vi "tcpMessageClient.vi"(11 "client configuration":T2={"client ID"="tcpClient", "remote host"="localhost", "local port"=50000, "remote port"=50001}) -> (0 "error out":errorcluster)   [LabVIEW 2014]
doc: "A couple tcpMessageServer and tcpMessageClient ensures communication between two instances. Each one can both transmit or receive CR/LF terminated message strings; however one of the member has to be a Server and the other a Client. Both sit and wait for the other party to connect.\n\nThe difference is: \n* the Server accpts connections on the specified port from any incoming host (the inputs \"remote host\" and \"remote port\" are ignored) \n* the Client must know to which host is directed\n\nCommunication with them, while running, is done via four named queues. One acts as a transmission buffer, another as a receive buffer; one is a single element queue, which cause the shutdown of the actor when a True is enqueued to it; the last one is a read only one-element queue which reports the actor status."
uses:
  typedefs/clientConfiguration.ctl
  typedefs/clientStatus.ctl
panel:
  out "status":T1
  out "received string":string
  out "string to send":string
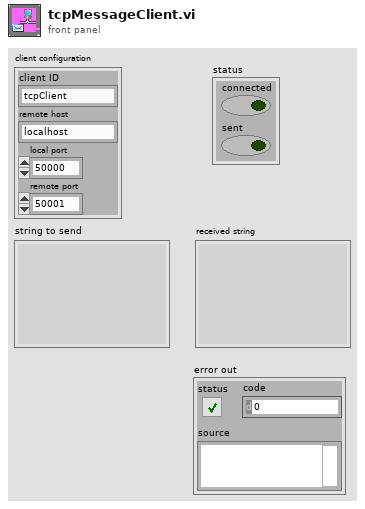
[diagram p1: front panel]
types:
  T1 = typedef "clientStatus.ctl" = cluster{"connected":bool, "sent":bool}
  T2 = typedef "clientConfiguration.ctl" = cluster{"client ID":string, "remote host":string, "local port":u16, "remote port":u16}
  T3 = cluster{"status":cluster{"queue":refnum<queue>, "error out":errorcluster}, "receive":cluster{"queue":refnum<queue>, "error out":errorcluster}, "transmit":cluster{"queue":refnum<queue>, "error out":errorcluster}, "shutdown":cluster{"queue":refnum<queue>, "error out":errorcluster}}
  T4 = cluster{"queue":refnum<queue>, "error out":errorcluster}
  T5 = enum16{"Standard", "Buffered", "CRLF", "Immediate"}
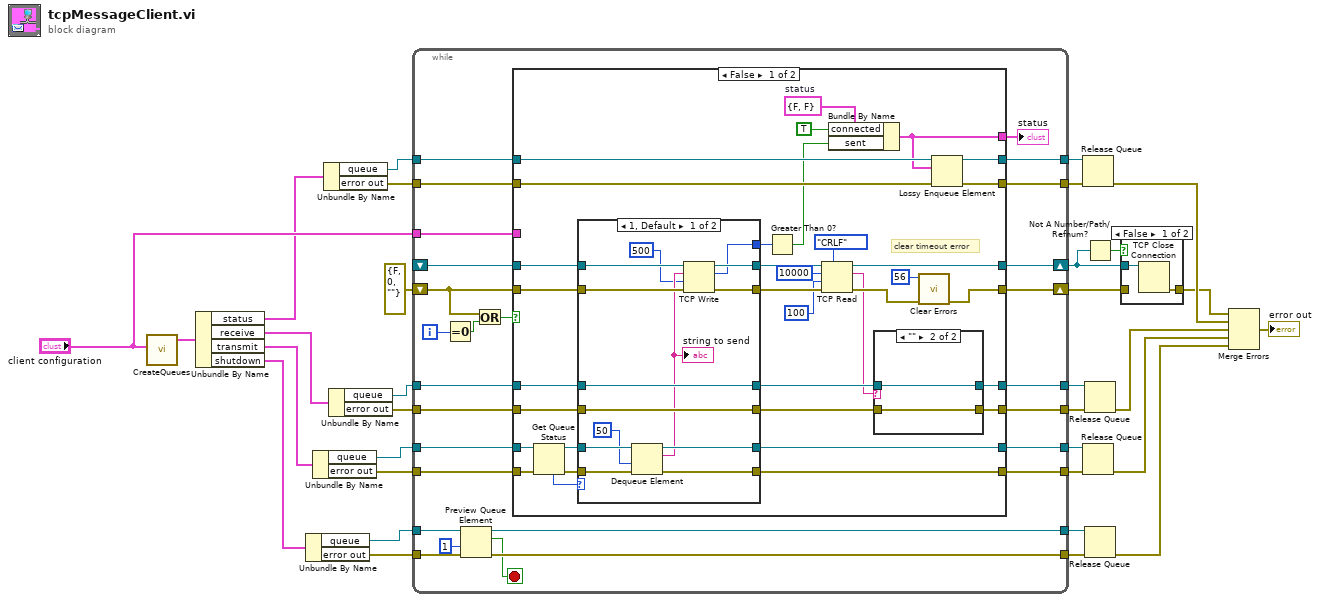
[diagram p0: block diagram]
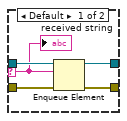
[diagram p3: hidden frame]
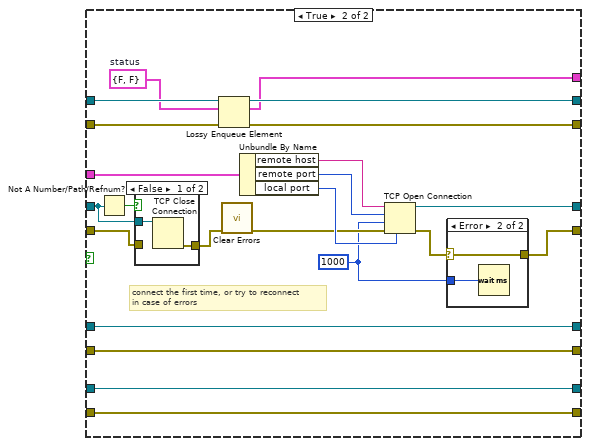
[diagram p5: hidden frame]
diagram:
  n1 = call "CreateQueues.vi"("client configuration"="client configuration") -> ("output cluster"=w5:T3)  [unwired: 10 in]
  n2 = Unbundle By Name(w5) -> ("status"=w8:T4, "receive"=w11:T4, "transmit"=w12:T4, "shutdown"=w17:T4)
  n3 = Unbundle By Name(w17) -> ("queue"=w16:refnum<queue>, "error out"=w15:errorcluster)
  n4 = Unbundle By Name(w12) -> ("queue"=w13:refnum<queue>, "error out"=w14:errorcluster)
  n5 = Unbundle By Name(w8) -> ("queue"=w7:refnum<queue>, "error out"=w6:errorcluster)
  n6 = Unbundle By Name(w11) -> ("queue"=w10:refnum<queue>, "error out"=w9:errorcluster)
  n7 = while {
    shift-right: [w57] -> w2
    shift-left: errorcluster {"status"=FALSE, "code"=0, "source"=""} ("error out") -> [w56]
    shift-right: [w58] -> w3
    shift-left: _ -> [w59]
    tunnel: "client configuration" -> [w52]
    tunnel: w15 -> [w37]
    tunnel: w16 -> [w38]
    tunnel: w7 -> [w51]
    tunnel: w6 -> [w50]
    tunnel: w10 -> [w49]
    tunnel: w9 -> [w48]
    tunnel: w13 -> [w47]
    tunnel: w14 -> [w46]
    tunnel: [w36] -> w31
    tunnel: [w35] -> w30
    tunnel: [w45] -> w29
    tunnel: [w44] -> w28
    tunnel: [w42] -> w27
    tunnel: [w41] -> w26
    tunnel: [w40] -> w25
    tunnel: [w39] -> w24
    i -> [w55]
    stop <- w33 stop-if-true
    n8 = Equal To 0?(x=w55) -> (x = 0?=w54:bool)
    n9 = Preview Queue Element(queue=w38, timeout in ms (-1)=1, error in (no error)=w37) -> (queue out=w36:refnum<queue>, element=w33:bool, error out=w35:errorcluster)  [unwired: 1 out]
    n10 = Or(x=w56, y=w54) -> (x .or. y?=w53:bool)
    n11 = case shown="False" w53 {
      tunnel: w59 -> [w77 w126]
      tunnel: [w72 w138] -> w58
      tunnel: [w67 w122] -> w57
      tunnel: w56 -> [w76 w125]
      tunnel: w52 -> [_ w141]
      tunnel: w51 -> [w93 w137]
      tunnel: w50 -> [w92 w136]
      tunnel: w49 -> [w79 w132]
      tunnel: w48 -> [w78 w131]
      tunnel: w47 -> [w87 w130]
      tunnel: w46 -> [w86 w129]
      tunnel: [w91 w135] -> w45
      tunnel: [w90 w134] -> w44
      tunnel: [w82 w133] -> w43
      tunnel: [w64 w132] -> w42
      tunnel: [w63 w131] -> w41
      tunnel: [w81 w130] -> w40
      tunnel: [w80 w129] -> w39
      frame False {
        w89 = T1 {"connected"=FALSE, "sent"=FALSE}  # status
        # "clear timeout error"
        n12 = Get Queue Status(queue=w87, error in (no error)=w86) -> (queue out=w84:refnum<queue>, error out=w83:errorcluster, # elements in queue=w85:i32)  [unwired: 1 in, 5 out]
        n13 = case shown="1, Default" w85 {
          tunnel: w84 -> [w114 w116]
          tunnel: w83 -> [w113 w115]
          tunnel: [w112 w116] -> w81
          tunnel: [w111 w115] -> w80
          tunnel: w79 -> [w110 w120]
          tunnel: w78 -> [w109 w119]
          tunnel: [w110 w120] -> w66
          tunnel: [w109 w119] -> w65
          tunnel: w77 -> [w108 w118]
          tunnel: w76 -> [w107 w117]
          tunnel: [w106 w118] -> w75
          tunnel: [w105 w117] -> w71
          tunnel: [w104 _] -> w74
          frame 1, Default {
            n14 = Dequeue Element(queue=w114, timeout in ms (-1)=50, error in (no error)=w113) -> (queue out=w112:refnum<queue>, element=w103:string, error out=w111:errorcluster)  [unwired: 1 out]
            "string to send" <- w103
            n15 = TCP Write(connection ID=w108, data in=w103, error in (no error)=w107, 9:500 ("timeout ms (25000)")) -> (connection ID out=w106:refnum<k5>, bytes written=w104:i32, error out=w105:errorcluster)
          }
          frame 0 {
          }
        }
        n16 = Greater Than 0?(x=w74) -> (x > 0?=w73:bool)
        n17 = TCP Read(connection ID=w75, bytes to read=10000, error in (no error)=w71, 7:T5."CRLF" ("mode (standard)"), 9:100 ("timeout ms (25000)")) -> (connection ID out=w72:refnum<k5>, data out=w62:string, error out=w70:errorcluster)
        n18 = Bundle By Name(cluster=w89, "connected"=TRUE, "sent"=w73) -> (w82:T1)
        n19 = case shown="\"\"" w62 {
          selector: w62 -> [w94 _]
          tunnel: w66 -> [w96 w100]
          tunnel: w65 -> [w95 w99]
          tunnel: [w98 w100] -> w64
          tunnel: [w97 w99] -> w63
          frame Default {
            n20 = Enqueue Element(queue=w96, element=w94, error in (no error)=w95) -> (queue out=w98:refnum<queue>, error out=w97:errorcluster)  [unwired: 1 in, 1 out]
            "received string" <- w94
          }
          frame "" {
          }
        }
        n21 = call <vilib>:"Clear Errors.vi"("error in (no error)"=w70, "specific error code to clear (0: all)"=56) -> ("error out"=w67:errorcluster)  [unwired: 4 in, 1 out]
        n22 = Lossy Enqueue Element(queue=w93, element=w82, error in (no error)=w92) -> (queue out=w91:refnum<queue>, error out=w90:errorcluster)  [unwired: 2 out]
      }
      frame True {
        w133 = T1 {"connected"=FALSE, "sent"=FALSE}  # status
        w121 = 1000 ("timeout ms (60000)")
        # "connect the first time, or try to reconnect\nin case of errors"
        n23 = Not A Number/Path/Refnum?(number/path/refnum=w126) -> (NaN/Path/Refnum?=w127:bool)
        n24 = case shown="False" w127 {
          tunnel: w126 -> [w147 _]
          tunnel: w125 -> [_ w148]
          tunnel: [w146 w148] -> w124
          frame False {
            n25 = TCP Close Connection(connection ID=w147) -> (error out=w146:errorcluster)  [unwired: 2 in, 1 out]
          }
          frame True {
          }
        }
        n26 = Lossy Enqueue Element(queue=w137, element=w133, error in (no error)=w136) -> (queue out=w135:refnum<queue>, error out=w134:errorcluster)  [unwired: 2 out]
        n27 = call <vilib>:"Clear Errors.vi"("error in (no error)"=w124) -> ("error out"=w128:errorcluster)  [unwired: 5 in, 1 out]
        n28 = Unbundle By Name(w141) -> ("remote host"=w140:string, "remote port"=w142:u16, "local port"=w139:u16)
        n29 = TCP Open Connection(address=w140, remote port or service name=w142, timeout ms (60000)=w121, local port=w139, error in (no error)=w128) -> (connection ID=w138:refnum<k5>, error out=w123:errorcluster)
        n30 = case shown="Error" w123 {
          selector: w123 -> [w143 w145]
          tunnel: [w143 w145] -> w122
          tunnel: w121 -> [_ w144]
          frame No Error {
          }
          frame Error {
            n31 = Wait (ms)(milliseconds to wait=w144) -> ()  [unwired: 1 out]
          }
        }
      }
    }
    "status" <- w43
  }
  n32 = Release Queue(queue=w29, error in (no error)=w28) -> (error out=w23:errorcluster)  [unwired: 1 in, 2 out]
  n33 = Release Queue(queue=w25, error in (no error)=w24) -> (error out=w21:errorcluster)  [unwired: 1 in, 2 out]
  n34 = Not A Number/Path/Refnum?(number/path/refnum=w3) -> (NaN/Path/Refnum?=w4:bool)
  n35 = Release Queue(queue=w27, error in (no error)=w26) -> (error out=w22:errorcluster)  [unwired: 1 in, 2 out]
  n36 = Release Queue(queue=w31, error in (no error)=w30) -> (error out=w20:errorcluster)  [unwired: 1 in, 2 out]
  n37 = case shown="False" w4 {
    tunnel: w3 -> [w150 _]
    tunnel: w2 -> [_ w151]
    tunnel: [w149 w151] -> w1
    frame False {
      n38 = TCP Close Connection(connection ID=w150) -> (error out=w149:errorcluster)  [unwired: 2 in, 1 out]
    }
    frame True {
    }
  }
  n39 = Merge Errors(w1, w23, w22, w21, w20) -> (→"error out":errorcluster)
